vi "Some DVR Method.vi"(0 "Session Handle in":T1, 11 "error in (no error)":errorcluster) -> (4 "Session Handle out":T1, 15 "error out":errorcluster)   [LabVIEW 2020, in "HTS.lvlib" / "Engine.lvclass"]
uses:
  Engine.lvclass
  Typedefs/Session Handle.ctl
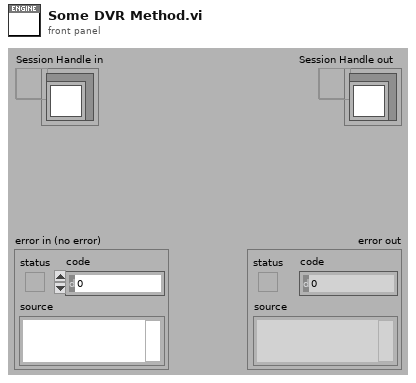
[diagram p1: front panel]
types:
  T1 = typedef "HTS.lvlib/Engine.lvclass/Session Handle.ctl" = refnum<data-value>
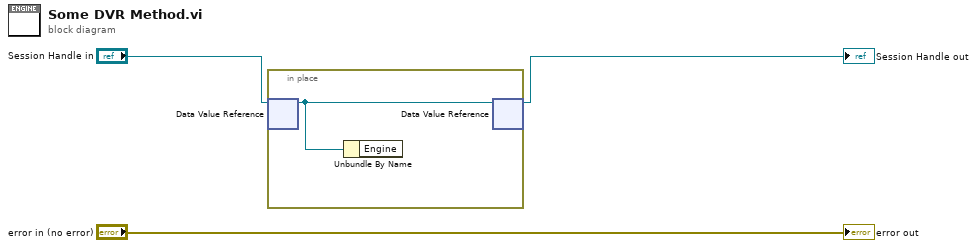
[diagram p0: block diagram]
diagram:
  n1 = in-place {
    n2 = in-place-dvr #1("Session Handle in") -> (w4:refnum<class "Engine.lvclass">)  [unwired: 1 out]
    n3 = Unbundle By Name(w4) -> ()  [unwired: 1 out]
    n4 = in-place-dvr #1(w4) -> (→"Session Handle out":T1)  [unwired: 1 out]
  }
  "error out" <- "error in (no error)"
